vi "Untitled 5.vi"(8 "error in (no error)":errorcluster, 11 "SignalMember in":refnum<class "SignalMember.lvclass">) -> (0 "error out":errorcluster, 3 "SignalMember out":refnum<class "SignalMember.lvclass">)   [LabVIEW 2011, in "SignalMember.lvclass"]
uses:
  SignalMember.lvclass
  SignalMember.lvclass/SignalMember.ctl
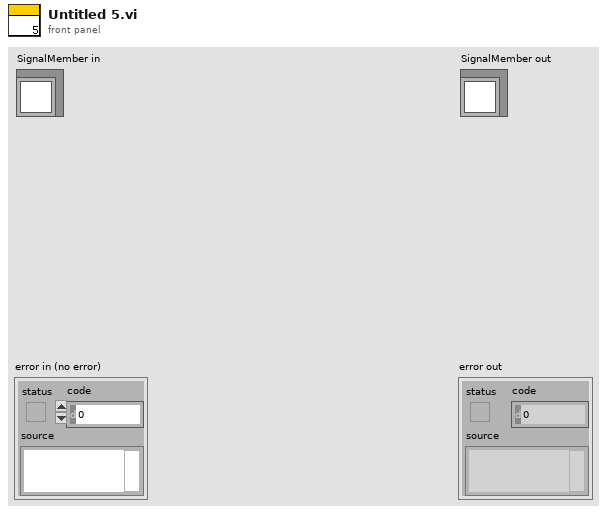
[diagram p1: front panel]
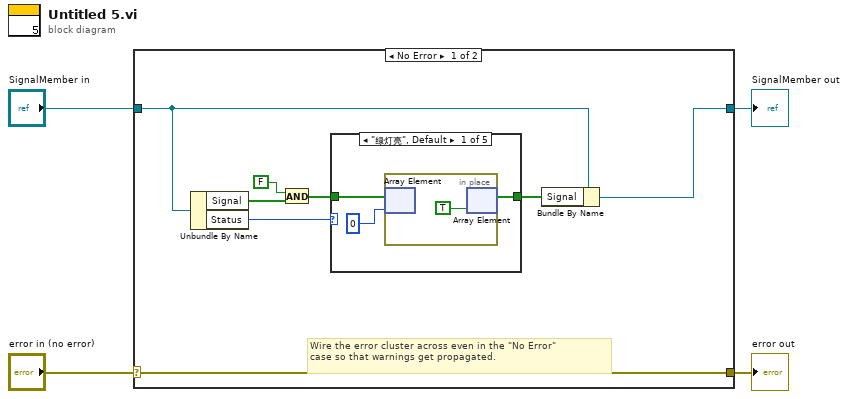
[diagram p0: block diagram]
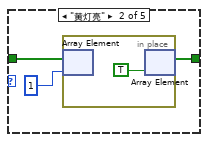
[diagram p2: hidden frame]
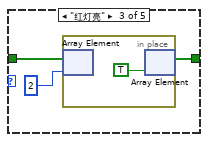
[diagram p3: hidden frame]
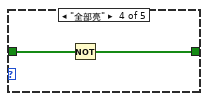
[diagram p4: hidden frame]
diagram:
  n1 = case shown="No Error" "error in (no error)" {
    selector: "error in (no error)" -> [w12 w29]
    tunnel: [w12 w29] -> w3
    tunnel: [w5 w28] -> w1
    tunnel: "SignalMember in" -> [w6 w28]
    frame No Error {
      # "Wire the error cluster across even in the \"No Error\"\ncase so that warnings get propagated."
      n2 = Unbundle By Name(w6) -> ("Signal"=w9:bool[], "Status"=w11:enum16{"绿灯亮", "黄灯亮", "红灯亮", "全部亮", "全部熄灭"})
      n3 = And(x=FALSE, y=w9) -> (x .and. y?=w10:bool[])
      n4 = case shown="\"绿灯亮\", Default" w11 {
        tunnel: w10 -> [w15 w19 w23 w26 w27]
        tunnel: [w13 w17 w21 w25 w27] -> w7
        frame "绿灯亮", Default {
          n5 = in-place {
            n6 = in-place-array #1(w15, 0) -> ()  [unwired: 1 out]
            n7 = in-place-array #1(TRUE ("element")) -> (w13:bool[])  [unwired: 1 out]
          }
        }
        frame "黄灯亮" {
          n8 = in-place {
            n9 = in-place-array #2(w19, 1) -> ()  [unwired: 1 out]
            n10 = in-place-array #2(TRUE ("element")) -> (w17:bool[])  [unwired: 1 out]
          }
        }
        frame "红灯亮" {
          n11 = in-place {
            n12 = in-place-array #3(w23, 2) -> ()  [unwired: 1 out]
            n13 = in-place-array #3(TRUE ("element")) -> (w21:bool[])  [unwired: 1 out]
          }
        }
        frame "全部亮" {
          n14 = Not(x=w26) -> (.not. x?=w25:bool[])
        }
        frame "全部熄灭" {
        }
      }
      n15 = Bundle By Name(cluster=w6, "Signal"=w7) -> (w5:refnum<class "SignalMember.lvclass">)
    }
    frame Error {
    }
  }
  "error out" <- w3
  "SignalMember out" <- w1
